vi "CalPSv2.vi"(0 "method":T2=1 items=["Least Square", "Least Absolute Residual", "Bisquare"], 4 "algorithm":T1=5 items=["SVD", "Givens", "Givens2", "Householder", "LU Decomposition", "Cholesky", "SVD for Rank Deficient H"], 6 "polynomial order (4)":i32=4, 8 "Stabilization Time (s) (6)":dbl=6.0, 9 "Field Points (101)":dbl=101.0, 10 "Gaussmeter GPIB Address":string="12", 11 "PS GPIB Address":string="1") -> (2 "Max Field (Oe)":dbl, 3 "Polynomial Coefficients":dbl[](array[numeric]))   [LabVIEW 2015]
doc: "Calibrates power supply output. Returns 4th order polynomial. Power Supply Output is result of polynomial as a function of field."
uses:
  <vilib>/Analysis/6fits.llb/Curve Fitting Criteria.ctl
  <vilib>/Analysis/6fits.llb/General Linear Fit Algorithm.ctl
  <vilib>/Analysis/NI_AALPro.lvlib
panel:
  out "PS Output":dbl
  out "Field (Oe)":dbl
  in  "Done":bool
  out "XY Graph":T3(graph)
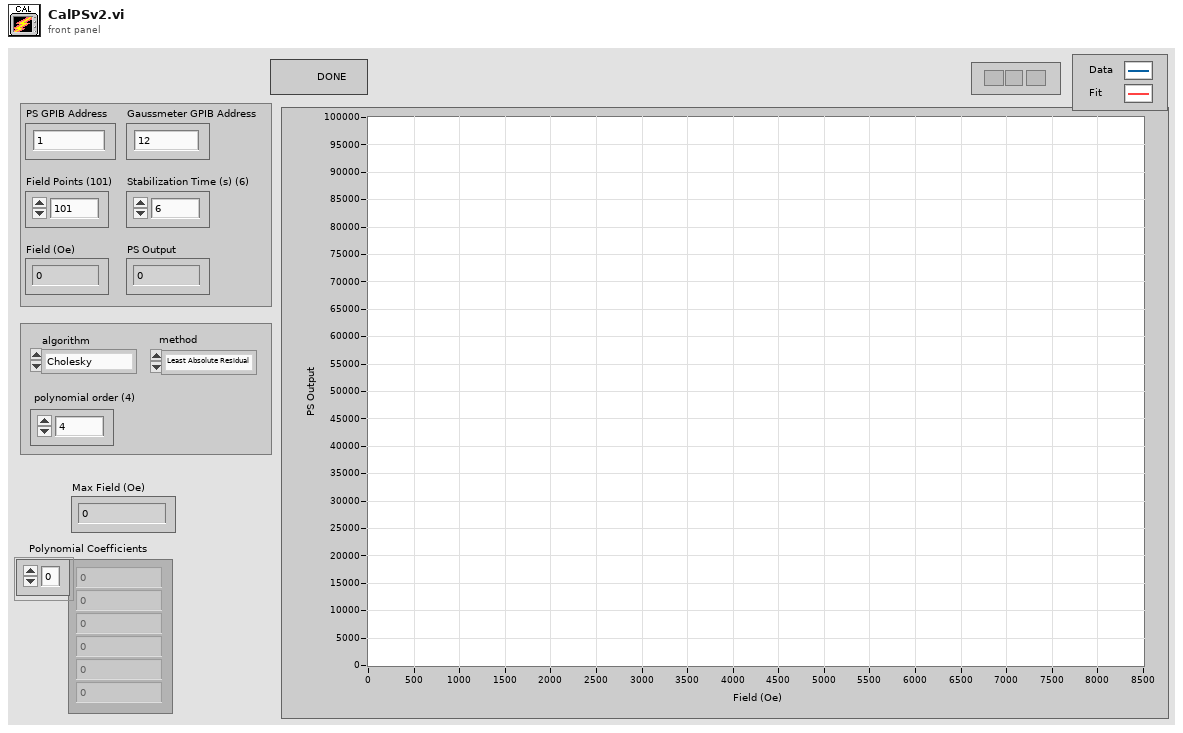
[diagram p1: front panel]
types:
  T1 = typedef "NI_AALPro.lvlib/General Linear Fit Algorithm.ctl" = u16
  T2 = typedef "NI_AALPro.lvlib/Curve Fitting Criteria.ctl" = u16
  T3 = cluster{"Field":dbl[], "Best Polynomial Fit":dbl[]}[]
  T4 = cluster{"Field":dbl[], "Best Polynomial Fit":dbl[]}
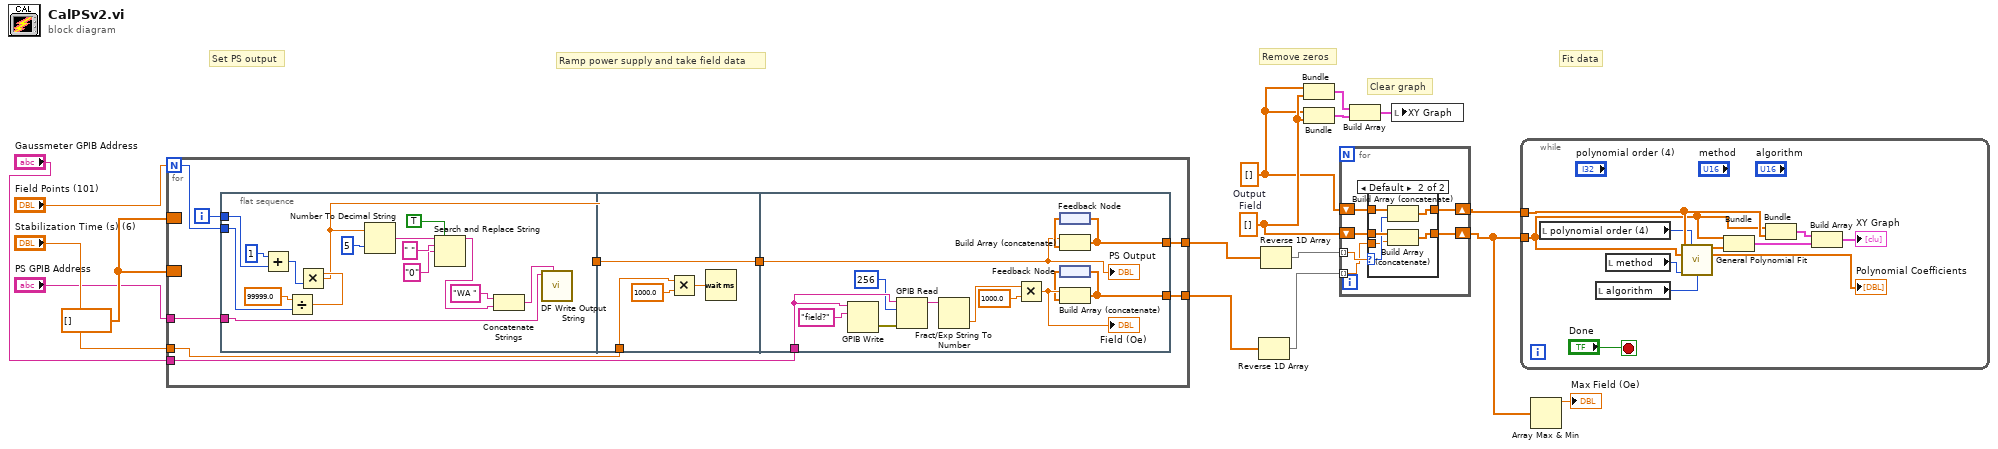
[diagram p0: block diagram]
diagram:
  w9 = dbl[] []
  w4 = dbl[] []  # Output
  w5 = dbl[] []  # Field
  # "Clear graph"
  # "Fit data"
  # "Set PS output"
  # "Ramp power supply and take field data"
  # "Remove zeros"
  n1 = for {
    N: "Field Points (101)" -> [w25]
    tunnel: "Gaussmeter GPIB Address" -> [w26]
    tunnel: "PS GPIB Address" -> [w18]
    tunnel: "Stabilization Time (s) (6)" -> [w23]
    border: w9 -> [_]
    border: w9 -> [_]
    tunnel: [w22] -> w8
    tunnel: [w21] -> w7
    i -> [w24]
    n2 = flat-sequence {
      tunnel: w18 -> [w42]
      tunnel: w25 -> [w38]
      tunnel: w24 -> [w35]
      tunnel: [w33] -> w19
      tunnel: w23 -> [w44]
      tunnel: [w43] -> w20
      tunnel: w19 -> [w43]
      tunnel: w26 -> [w59]
      tunnel: [w49] -> w21
      tunnel: [w51] -> w22
      tunnel: w20 -> [w47]
      frame #0 {
        n3 = Add(x=1, y=w35) -> (x+y=w36:i32)
        n4 = Divide(x=99999.0, y=w38) -> (x/y=w37:dbl)
        n5 = Multiply(x=w37, y=w36) -> (x*y=w33:dbl)
        n6 = Number To Decimal String(number=w33, width (-)=i16 5) -> (decimal integer string=w31:string)
        n7 = Search and Replace String(replace all?=TRUE ("replace all? (F)"), input string=w31, search string=" ", replace string="0" ("replace string (\"\")")) -> (result string=w28:string)  [unwired: 4 in, 3 out]
        n8 = Concatenate Strings("WA " ("string"), w28) -> (w40:string)
        n9 = call "DF Write Output String"("Write String"=w40, "GPIB Address"=w42) -> ()  [unwired: 7 in]
      }
      frame #1 {
        n10 = Multiply(x=w44, y=1000.0) -> (x*y=w46:dbl)
        n11 = Wait (ms)(milliseconds to wait=w46) -> ()  [unwired: 1 out]
      }
      frame #2 {
        n12 = GPIB Write(0:w59, 1:"field?" ("data")) -> (6:w55:errorcluster)  [unwired: 3 in, 1 out]
        n13 = GPIB Read(0:w59, 1:256 ("byte count"), 3:w55) -> (5:w56:string)  [unwired: 2 in, 2 out]
        n14 = Fract/Exp String To Number(string=w56) -> (number=w54:dbl)  [unwired: 3 in, 1 out]
        n15 = Multiply(x=w54, y=1000.0) -> (x*y=w52:dbl)
        "Field (Oe)" <- w52
        n16 = feedback #1() -> (w50:dbl[])
        n17 = Build Array (concatenate)(w47, w50) -> (w51:dbl[])
        n18 = feedback-in #1(w51) -> ()
        n19 = feedback #2() -> (w48:dbl[])
        n20 = Build Array (concatenate)(w52, w48) -> (w49:dbl[])
        n21 = feedback-in #2(w49) -> ()
        "PS Output" <- w47
      }
    }
  }
  n22 = Reverse 1D Array(array=w7) -> (reversed array=w12:dbl[])
  n23 = Reverse 1D Array(array=w8) -> (reversed array=w13:dbl[])
  n24 = Bundle("Output"=w4, "Field"=w5) -> (w3:cluster{"Output":dbl[], "Field":dbl[]})  [unwired: 1 in]
  n25 = Bundle("Output"=w4, "Field"=w5) -> (w2:cluster{"Output":dbl[], "Field":dbl[]})  [unwired: 1 in]
  n26 = for {
    tunnel: w12 -> [w61] mode=indexing
    shift-right: [w65] -> w15
    shift-left: w5 -> [w64]
    shift-right: [w60] -> w14
    shift-left: w4 -> [w63]
    tunnel: w13 -> [w62] mode=indexing
    n27 = case shown="Default" w62 {
      selector: w62 -> [_ w71]
      tunnel: w64 -> [w67 w73]
      tunnel: [w67 w72] -> w65
      tunnel: w63 -> [w66 w68]
      tunnel: w61 -> [_ w70]
      tunnel: [w66 w69] -> w60
      frame 0 {
      }
      frame Default {
        n28 = Build Array (concatenate)(w68, w71) -> (w69:dbl[])
        n29 = Build Array (concatenate)(w73, w70) -> (w72:dbl[])
      }
    }
  }
  n30 = Build Array(w3, w2) -> (w1:cluster{"Output":dbl[], "Field":dbl[]}[])
  n31 = local write "XY Graph"(w1) -> ()
  n32 = while {
    tunnel: w14 -> [w84]
    tunnel: w15 -> [w74]
    stop <- "Done" stop-if-true
    n33 = local read "polynomial order (4)"() -> (w79:i32)
    n34 = local read "algorithm"() -> (w77:T1)
    n35 = local read "method"() -> (w78:T2)
    n36 = call <vilib>:"General Polynomial Fit.vi"("Y"=w84, "polynomial order"=w79, "X"=w74, "method"=w78, "algorithm"=w77) -> ("Best Polynomial Fit"=w80:dbl[], "Polynomial Coefficients"=→"Polynomial Coefficients":dbl[])  [unwired: 7 in, 2 out]
    n37 = Bundle("Field"=w74, "Best Polynomial Fit"=w80) -> (w81:T4)  [unwired: 1 in]
    n38 = Bundle("Field"=w74, "Output"=w84) -> (w82:cluster{"Field":dbl[], "Output":dbl[]})  [unwired: 1 in]
    n39 = Build Array(w82, w81) -> (→"XY Graph":T3)
  }
  n40 = Array Max & Min(array=w15) -> (max value=→"Max Field (Oe)":dbl)  [unwired: 3 out]
